vi "Update Counter Controls.vi"(8 "error in (no error)":errorcluster, 10 "SD Control Refs in":T6, 11 "Counter Channel":T1={"Measurement Mode"=0, "Count Edges"={"Counter Event"=0, "Counter Source"=0, "Counter Direction"=0, "Terminal Count"=4294967295, "Output Mode"=0, "Gate Mode"=3}, "Period Measurement"={"Measurement Edge"=0}, "Pulse Width Measurement"={"Measurement Type"=3}, "Frequency Measurement"={"Measurement Edge"=0, "Measurement Timebase"=0}} {"Frequency Measurement"."Measurement Timebase" items=["256 us", "512 us", "1024 us", "2048 us", "4096 us", "8192 us", "16384 us", "32768 us"]; "Frequency Measurement"."Measurement Edge" items=["Rising Edge", "Falling Edge"]; "Pulse Width Measurement"."Measurement Type" items=["High Pulse"=3, "Low Pulse"=4, "Most Recent"=5]; "Period Measurement"."Measurement Edge" items=["Rising Edge", "Falling Edge"]; "Count Edges"."Gate Mode" items=["Next Channel"=1, "Always Enabled"=3]; "Count Edges"."Output Mode" items=["Toggle, Reset Off", "Toggle, Reset On", "On Pulse", "Off Pulse"]; "Count Edges"."Counter Direction" items=["Count up", "Count down"]; "Count Edges"."Counter Source" items=["This Channel", "Terminal count of previous channel"]; "Count Edges"."Counter Event" items=["Rising Edge", "Falling Edge", "Any Edge"]; "Measurement Mode" items=["Count Edges", "Period Measurements", "Pulse Width Measurements", "Frequency Measurements"]}) -> (0 "error out":errorcluster)   [LabVIEW 2017, in "Modules.lvlib" / "SD Module.lvclass"]
uses:
  SD Module.lvclass
  Type Defs/SD Control Refs.ctl
  Type Defs/Main Control Refs.ctl
  Type Defs/Counter Control Refs.ctl
  Type Defs/CDO Control Refs.ctl
  Type Defs/PWM Control Refs.ctl
  Type Defs/Quadrature Control Refs.ctl
  Type Defs/Counter Channel.ctl
  Type Defs/Count Edges.ctl
  Type Defs/Period Measurement.ctl
  Type Defs/Pulse Width Measurement.ctl
  Type Defs/Frequency Measurement.ctl
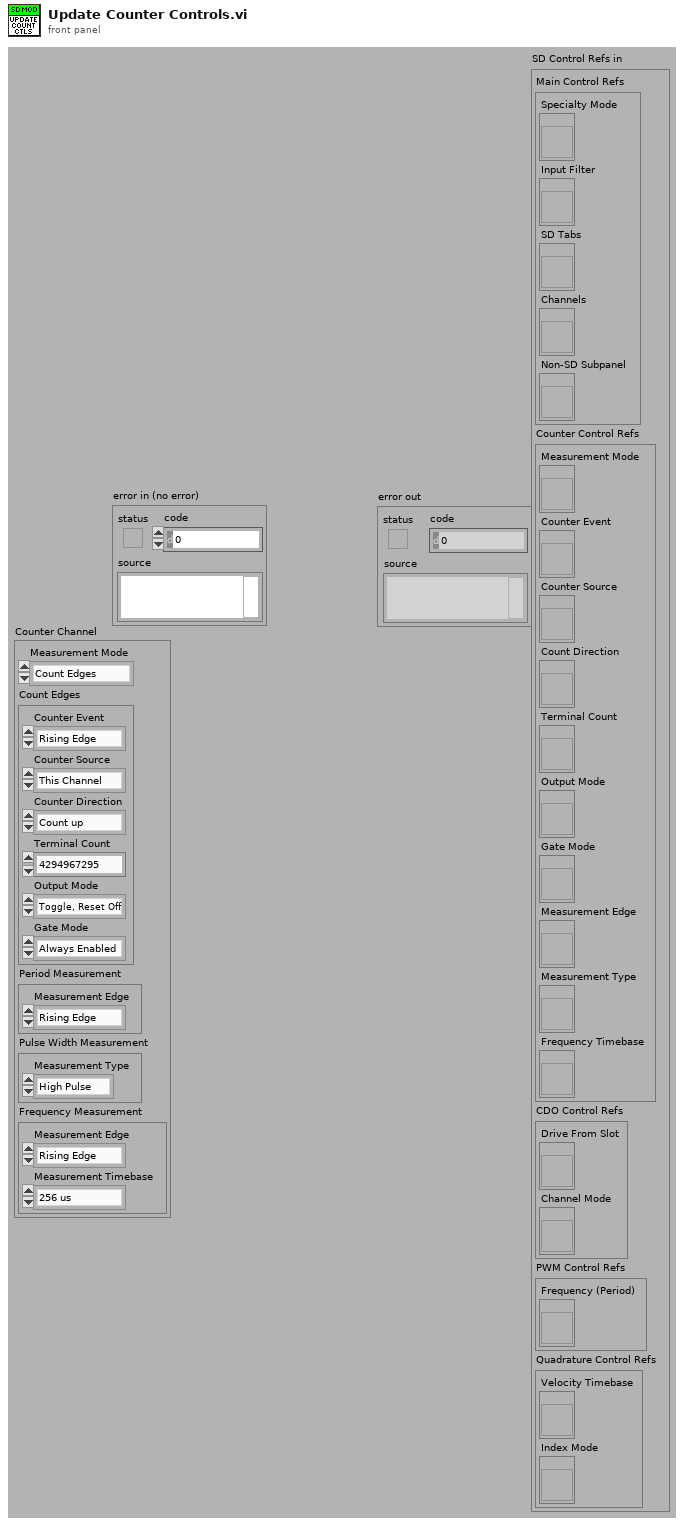
[diagram p1: front panel]
types:
  T1 = typedef "Modules.lvlib/SD Module.lvclass/Counter Channel.ctl" = cluster{"Measurement Mode":u32, "Count Edges":T2, "Period Measurement":T3, "Pulse Width Measurement":T4, "Frequency Measurement":T5}
  T2 = typedef "Modules.lvlib/SD Module.lvclass/Count Edges.ctl" = cluster{"Counter Event":u32, "Counter Source":u32, "Counter Direction":u32, "Terminal Count":u32, "Output Mode":u32, "Gate Mode":u32}
  T3 = typedef "Modules.lvlib/SD Module.lvclass/Period Measurement.ctl" = cluster{"Measurement Edge":u32}
  T4 = typedef "Modules.lvlib/SD Module.lvclass/Pulse Width Measurement.ctl" = cluster{"Measurement Type":u32}
  T5 = typedef "Modules.lvlib/SD Module.lvclass/Frequency Measurement.ctl" = cluster{"Measurement Edge":u32, "Measurement Timebase":u32}
  T6 = typedef "Modules.lvlib/SD Module.lvclass/SD Control Refs.ctl" = cluster{"Main Control Refs":T7, "Counter Control Refs":T8, "CDO Control Refs":T9, "PWM Control Refs":T10, "Quadrature Control Refs":T11}
  T7 = typedef "Modules.lvlib/SD Module.lvclass/Main Control Refs.ctl" = cluster{"Specialty Mode":refnum<vi>, "Input Filter":refnum<vi>, "SD Tabs":refnum<vi>, "Channels":refnum<vi>, "Non-SD Subpanel":refnum<vi>}
  T8 = typedef "Modules.lvlib/SD Module.lvclass/Counter Control Refs.ctl" = cluster{"Measurement Mode":refnum<vi>, "Counter Event":refnum<vi>, "Counter Source":refnum<vi>, "Count Direction":refnum<vi>, "Terminal Count":refnum<vi>, "Output Mode":refnum<vi>, "Gate Mode":refnum<vi>, "Measurement Edge":refnum<vi>, "Measurement Type":refnum<vi>, "Frequency Timebase":refnum<vi>}
  T9 = typedef "Modules.lvlib/SD Module.lvclass/CDO Control Refs.ctl" = cluster{"Drive From Slot":refnum<vi>, "Channel Mode":refnum<vi>}
  T10 = typedef "Modules.lvlib/SD Module.lvclass/PWM Control Refs.ctl" = cluster{"Frequency (Period)":refnum<vi>}
  T11 = typedef "Modules.lvlib/SD Module.lvclass/Quadrature Control Refs.ctl" = cluster{"Velocity Timebase":refnum<vi>, "Index Mode":refnum<vi>}
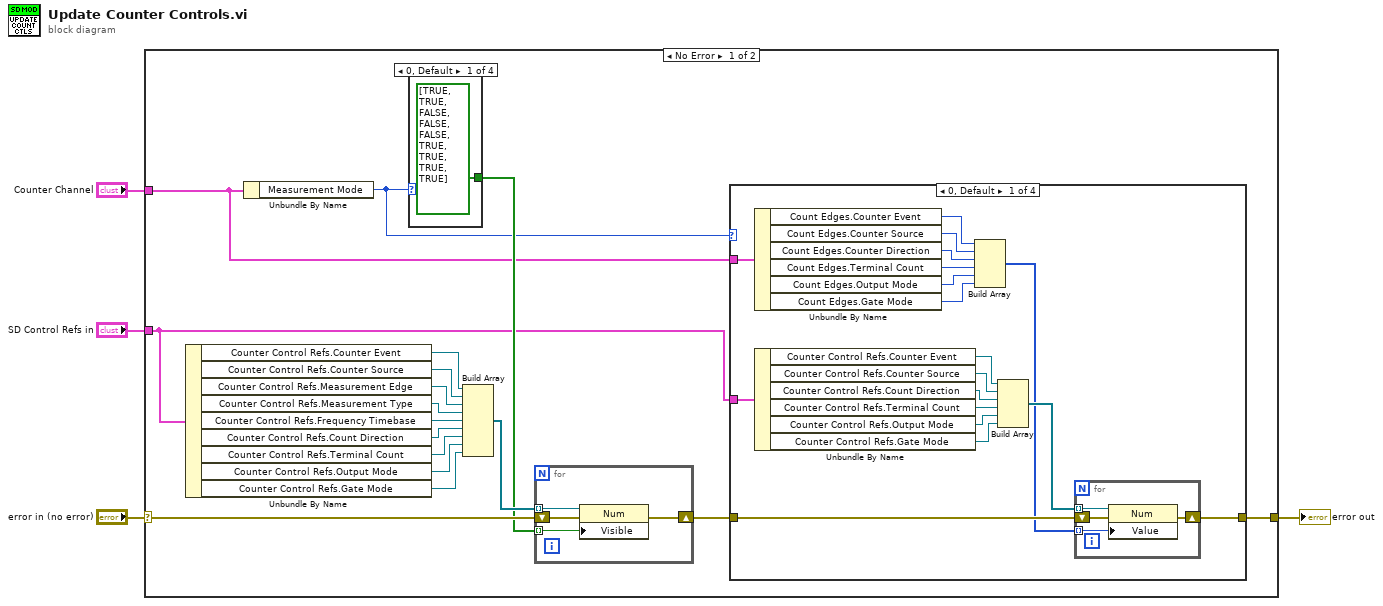
[diagram p0: block diagram]
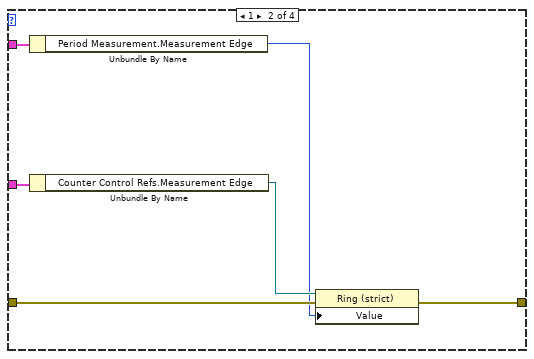
[diagram p2: hidden frame]
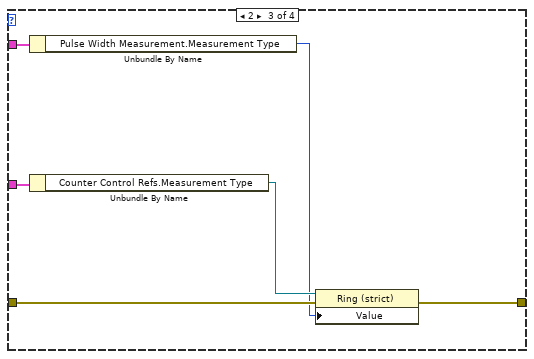
[diagram p3: hidden frame]
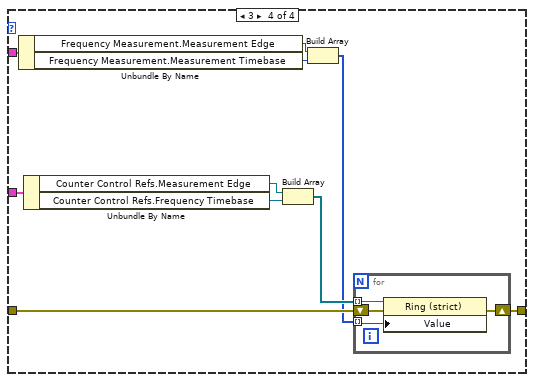
[diagram p4: hidden frame]
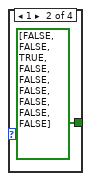
[diagram p5: hidden frame]
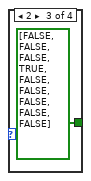
[diagram p6: hidden frame]
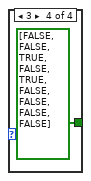
[diagram p7: hidden frame]
diagram:
  n1 = case shown="No Error" "error in (no error)" {
    selector: "error in (no error)" -> [w15 w78]
    tunnel: [w9 w78] -> w3
    tunnel: "SD Control Refs in" -> [w11 _]
    tunnel: "Counter Channel" -> [w10 _]
    frame No Error {
      n2 = Unbundle By Name(w11) -> ("Counter Control Refs.Counter Event"=w17:refnum<vi>, "Counter Control Refs.Counter Source"=w20:refnum<vi>, "Counter Control Refs.Measurement Edge"=w21:refnum<vi>, "Counter Control Refs.Measurement Type"=w19:refnum<vi>, "Counter Control Refs.Frequency Timebase"=w18:refnum<vi>, "Counter Control Refs.Count Direction"=w8:refnum<vi>, "Counter Control Refs.Terminal Count"=w7:refnum<vi>, "Counter Control Refs.Output Mode"=w6:refnum<vi>, "Counter Control Refs.Gate Mode"=w5:refnum<vi>)
      n3 = Unbundle By Name(w10) -> ("Measurement Mode"=w13:u32)
      n4 = case shown="0, Default" w13 {
        tunnel: [bool[] [TRUE, TRUE, FALSE, FALSE, FALSE, TRUE, TRUE, TRUE, TRUE] bool[] [FALSE, FALSE, TRUE, FALSE, FALSE, FALSE, FALSE, FALSE, FALSE] bool[] [FALSE, FALSE, FALSE, TRUE, FALSE, FALSE, FALSE, FALSE, FALSE] bool[] [FALSE, FALSE, TRUE, FALSE, TRUE, FALSE, FALSE, FALSE, FALSE]] -> w14
        frame 0, Default {
        }
        frame 1 {
        }
        frame 2 {
        }
        frame 3 {
        }
      }
      n5 = Build Array(w17, w20, w21, w19, w18, w8, w7, w6, w5) -> (w16:refnum<vi>[])
      n6 = for {
        tunnel: w16 -> [w77] mode=indexing
        shift-right: [w75] -> w12
        shift-left: w15 -> [w76]
        tunnel: w14 -> [w74] mode=indexing
        n7 = property class="Num"(reference=w77, error in=w76, "Visible"=w74) -> (error out=w75:errorcluster)  [unwired: 1 out]
      }
      n8 = case shown="0, Default" w13 {
        tunnel: w12 -> [w31 w47 w53 w63]
        tunnel: w11 -> [w32 w48 w54 w64]
        tunnel: w10 -> [w39 w49 w55 w65]
        tunnel: [w22 w46 w52 w62] -> w9
        frame 0, Default {
          n9 = Unbundle By Name(w39) -> ("Count Edges.Counter Event"=w35:u32, "Count Edges.Counter Source"=w36:u32, "Count Edges.Counter Direction"=w37:u32, "Count Edges.Terminal Count"=w38:u32, "Count Edges.Output Mode"=w34:u32, "Count Edges.Gate Mode"=w33:u32)
          n10 = Unbundle By Name(w32) -> ("Counter Control Refs.Counter Event"=w29:refnum<vi>, "Counter Control Refs.Counter Source"=w28:refnum<vi>, "Counter Control Refs.Count Direction"=w27:refnum<vi>, "Counter Control Refs.Terminal Count"=w26:refnum<vi>, "Counter Control Refs.Output Mode"=w25:refnum<vi>, "Counter Control Refs.Gate Mode"=w24:refnum<vi>)
          n11 = Build Array(w35, w36, w37, w38, w34, w33) -> (w23:u32[])
          n12 = Build Array(w29, w28, w27, w26, w25, w24) -> (w30:refnum<vi>[])
          n13 = for {
            shift-right: [w42] -> w22
            shift-left: w31 -> [w43]
            tunnel: w30 -> [w41] mode=indexing
            tunnel: w23 -> [w40] mode=indexing
            n14 = property class="Num"(reference=w41, error in=w43, "Value"=w40) -> (error out=w42:errorcluster)  [unwired: 1 out]
          }
        }
        frame 1 {
          n15 = Unbundle By Name(w49) -> ("Period Measurement.Measurement Edge"=w44:u32)
          n16 = Unbundle By Name(w48) -> ("Counter Control Refs.Measurement Edge"=w45:refnum<vi>)
          n17 = property class="Ring (strict)"(reference=w45, error in=w47, "Value"=w44) -> (error out=w46:errorcluster)  [unwired: 1 out]
        }
        frame 2 {
          n18 = Unbundle By Name(w55) -> ("Pulse Width Measurement.Measurement Type"=w50:u32)
          n19 = Unbundle By Name(w54) -> ("Counter Control Refs.Measurement Type"=w51:refnum<vi>)
          n20 = property class="Ring (strict)"(reference=w51, error in=w53, "Value"=w50) -> (error out=w52:errorcluster)  [unwired: 1 out]
        }
        frame 3 {
          n21 = Unbundle By Name(w65) -> ("Frequency Measurement.Measurement Edge"=w58:u32, "Frequency Measurement.Measurement Timebase"=w59:u32)
          n22 = Unbundle By Name(w64) -> ("Counter Control Refs.Measurement Edge"=w60:refnum<vi>, "Counter Control Refs.Frequency Timebase"=w61:refnum<vi>)
          n23 = Build Array(w60, w61) -> (w57:refnum<vi>[])
          n24 = Build Array(w58, w59) -> (w56:u32[])
          n25 = for {
            shift-right: [w66] -> w62
            shift-left: w63 -> [w69]
            tunnel: w57 -> [w68] mode=indexing
            tunnel: w56 -> [w67] mode=indexing
            n26 = property class="Ring (strict)"(reference=w68, error in=w69, "Value"=w67) -> (error out=w66:errorcluster)  [unwired: 1 out]
          }
        }
      }
    }
    frame Error {
    }
  }
  "error out" <- w3
